vi "Draw_fixed_grid.vi"(7 "Grid Line Color":u32(colorbox)=16760386, 8 "error in (no error)":errorcluster, 9 "Grid name":string="grid2", 10 "Grid Lines":u32=2, 11 "Image In":T1) -> (0 "error out":errorcluster, 3 "Image Out":T1)   [LabVIEW 2020]
doc: "This example program overlays a grid on an image, displays it in an image display and writes a JPEG file with the grid overlay information. Follow the steps below to run the vi:\n\n1. Select an image file\n2. Select the spacing in pixels between grid lines\n3. Select the grid line color\n4. Run the VI"
uses:
  <vilib>/vision/Image Controls.llb/IMAQ Image.ctl
panel:
  out "nearest integer value 2":dbl
  out "nearest integer value":dbl
  out "Y Resolution":i32
  out "X Resolution":i32
  out "For Itr 2":i32
  out "For Itr1":i32
  out "Image":T1(plugin-control)
  out "Grid Line Spacing":u32=100
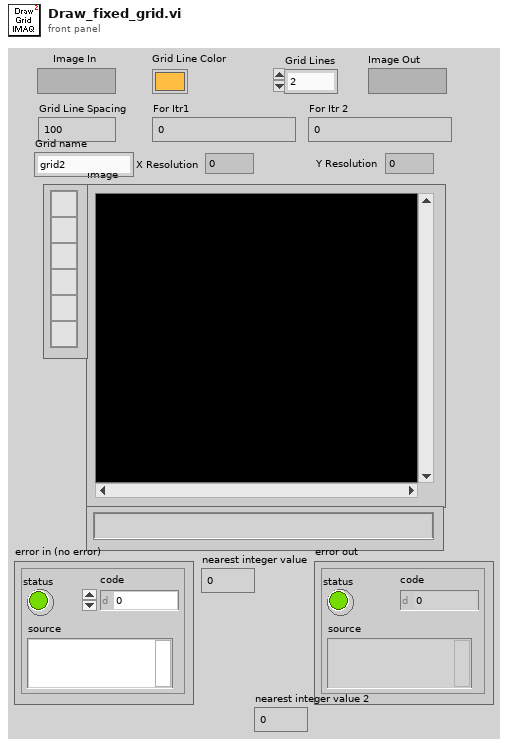
[diagram p1: front panel]
types:
  T1 = typedef "IMAQ Image.ctl" = refnum<image>
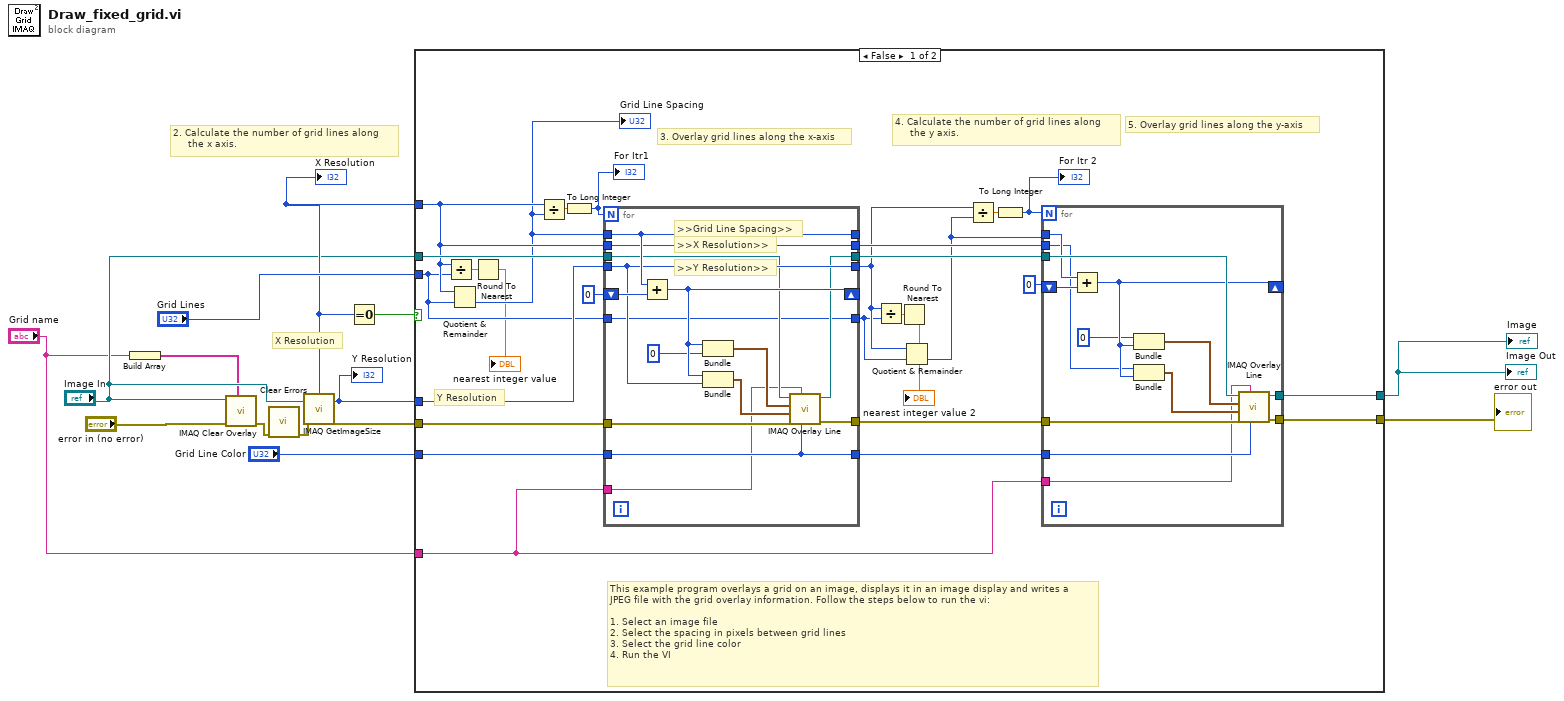
[diagram p0: block diagram]
diagram:
  # "X Resolution"
  # "2. Calculate the number of grid lines along\n     the x axis."
  n1 = Build Array("Grid name") -> (w2:string[])
  n2 = call "IMAQ Clear Overlay"("Groups"=w2, "error in (no error)"="error in (no error)", "Image"="Image In") -> ("error out"=w4:errorcluster)  [unwired: 7 in, 1 out]
  n3 = call <vilib>:"Clear Errors.vi"("error in (no error)"=w4) -> ("error out"=w3:errorcluster)  [unwired: 5 in, 1 out]
  n4 = call "IMAQ GetImageSize"("Image"="Image In", "error in (no error)"=w3) -> ("Y Resolution"=w13:i32, "X Resolution"=w7:i32, "error out"=w14:errorcluster)  [unwired: 2 in]
  "X Resolution" <- w7
  "Y Resolution" <- w13
  n5 = Equal To 0?(x=w7) -> (x = 0?=w6:bool)
  n6 = case shown="False" w6 {
    tunnel: w14 -> [w41 w70]
    tunnel: "Image In" -> [w39 w71]
    tunnel: w13 -> [w34 _]
    tunnel: "Grid Line Color" -> [w29 _]
    tunnel: [w27 w71] -> w11
    tunnel: [w26 w70] -> w10
    tunnel: w7 -> [w23 _]
    tunnel: "Grid Lines" -> [w22 _]
    tunnel: "Grid name" -> [w15 _]
    frame False {
      # "This example program overlays a grid on an image, displays it in an image display and writes a \nJPEG file with the grid overlay information. Follow the steps below to run the vi:\n\n1. Select an image file\n2. Select the spacing in pixels between grid lines\n3. Select the grid line color\n4. Run the VI"
      # "Y Resolution"
      # "5. Overlay grid lines along the y-axis"
      # "4. Calculate the number of grid lines along\n     the y axis."
      # "3. Overlay grid lines along the x-axis"
      n7 = Divide(x=w23, y=w22) -> (x/y=w25:dbl)
      n8 = Quotient & Remainder(x=w23, y=w22) -> (floor(x/y)=w21:u32)  [unwired: 1 out]
      "Grid Line Spacing" <- w21
      n9 = Round To Nearest(number=w25) -> (nearest integer value=→"nearest integer value":dbl)
      n10 = Divide(x=w23, y=w21) -> (x/y=w37:dbl)
      n11 = To Long Integer(number=w37) -> (32bit integer=w36:i32)
      "For Itr1" <- w36
      n12 = for {
        N: w36 -> [_]
        tunnel: w41 -> [w69]
        tunnel: [w68] -> w40
        tunnel: w39 -> [w57]
        tunnel: [w58] -> w38
        tunnel: w21 -> [w67]
        tunnel: [w67] -> _
        tunnel: [w63] -> w19
        tunnel: w34 -> [w63]
        shift-right: [w65] -> _
        shift-left: 0 -> [w66]
        tunnel: [w60] -> w31
        tunnel: w23 -> [w60]
        tunnel: w29 -> [w59]
        tunnel: [w59] -> w28
        tunnel: w22 -> [w56]
        tunnel: [w56] -> w18
        tunnel: w15 -> [w55]
        # ">>Y Resolution>>"
        # ">>X Resolution>>"
        # ">>Grid Line Spacing>>"
        n13 = Add(x=w67, y=w66) -> (x+y=w65:u32)
        n14 = Bundle(w65, 0) -> (w62:cluster{u32, i32})  [unwired: 1 in]
        n15 = Bundle(w65, "Y Resolution"=w63) -> (w61:cluster{u32, "Y Resolution":i32})  [unwired: 1 in]
        n16 = call "IMAQ Overlay Line"("Color"=w59, "Group"=w55, "error in (no error)"=w69, "End Point"=w61, "Start Point"=w62, "Image"=w57) -> ("error out"=w68:errorcluster, "Image Out"=w58:T1)  [unwired: 4 in]
      }
      n17 = Divide(x=w19, y=w18) -> (x/y=w24:dbl)
      n18 = Round To Nearest(number=w24) -> (nearest integer value=→"nearest integer value 2":dbl)
      n19 = Quotient & Remainder(x=w19, y=w18) -> (floor(x/y)=w16:u32)  [unwired: 1 out]
      n20 = Divide(x=w19, y=w16) -> (x/y=w35:dbl)
      n21 = To Long Integer(number=w35) -> (32bit integer=w30:i32)
      "For Itr 2" <- w30
      n22 = for {
        N: w30 -> [_]
        tunnel: w40 -> [w54]
        tunnel: [w53] -> w26
        tunnel: w38 -> [w52]
        shift-right: [w49] -> _
        shift-left: 0 -> [w51]
        tunnel: w16 -> [w50]
        tunnel: w31 -> [w47]
        tunnel: [w44] -> w27
        tunnel: w28 -> [w43]
        tunnel: w15 -> [w42]
        n23 = Add(x=w50, y=w51) -> (x+y=w49:u32)
        n24 = Bundle(0, w49) -> (w46:cluster{i32, u32})  [unwired: 1 in]
        n25 = Bundle("X Resolution"=w47, w49) -> (w45:cluster{"X Resolution":i32, u32})  [unwired: 1 in]
        n26 = call "IMAQ Overlay Line"("Color"=w43, "Group"=w42, "error in (no error)"=w54, "End Point"=w45, "Start Point"=w46, "Image"=w52) -> ("error out"=w53:errorcluster, "Image Out"=w44:T1)  [unwired: 4 in]
      }
    }
    frame True {
    }
  }
  "Image" <- w11
  "error out" <- w10
  "Image Out" <- w11
